vi "Write Preloaded Configuration.vi"(10 "Pre-Loaded Configuration":variant, 11 "TransientConfiguration in":refnum<class "TransientConfiguration.lvclass">) -> (3 "TransientConfiguration out":refnum<class "TransientConfiguration.lvclass">)   [LabVIEW 2020, in "TransientConfiguration.lvclass"]
uses:
  <vilib>/gpm_packages/@cs/Configuration/Source/TransientConfiguration/TransientConfiguration.lvclass
  <vilib>/gpm_packages/@cs/Configuration/Source/TransientConfiguration/TransientConfiguration.lvclass/TransientConfiguration.ctl
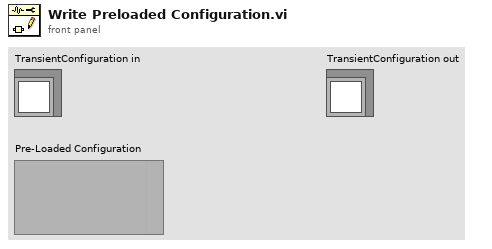
[diagram p1: front panel]
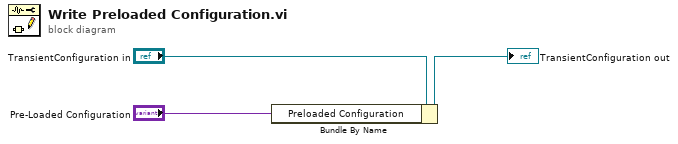
[diagram p0: block diagram]
diagram:
  n1 = Bundle By Name(cluster="TransientConfiguration in", "Preloaded Configuration"="Pre-Loaded Configuration") -> (→"TransientConfiguration out":refnum<class "TransientConfiguration.lvclass">)
